vi "Read commandName.vi"(8 "error in (no error)":errorcluster, 11 "GoToStandby in":refnum<class "SetSpectTempSetpoint.lvclass">) -> (0 "error out":errorcluster, 2 "CommandValue":T1, 3 "GoToStandby out":refnum<class "SetSpectTempSetpoint.lvclass">)   [LabVIEW 2016, in "Commands.lvlib" / "SetSpectTempSetpoint.lvclass"]
uses:
  SetSpectTempSetpoint.lvclass
  Typedefs/CommandValue.ctl
  Typedefs/EXATypedefs.lvlib
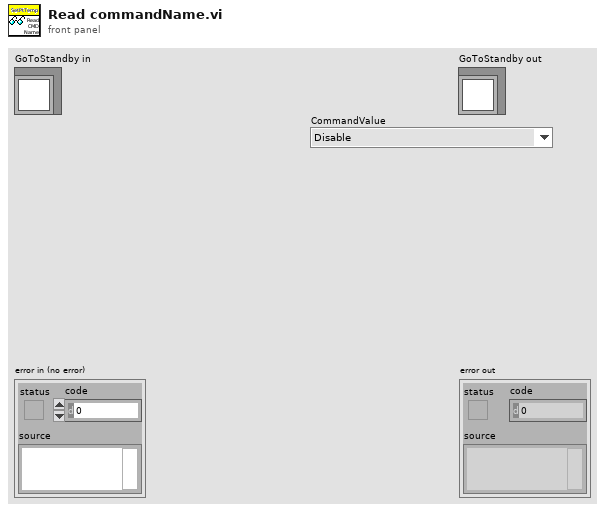
[diagram p1: front panel]
types:
  T1 = typedef "EXATypedefs.lvlib/CommandValue.ctl" = enum16{"Disable", "Enable", "Exit", "GoToStandby", "OnHeartbeat", "OnIncomingMessagingError", "OnInterrupt", "Start", "CaptureSpectImage", "SetSpectTempSetpoint", "StopImageCapture"}
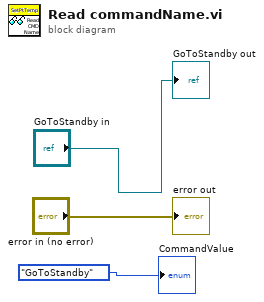
[diagram p0: block diagram]
diagram:
  "error out" <- "error in (no error)"
  "GoToStandby out" <- "GoToStandby in"
  "CommandValue" <- CommandValue."GoToStandby" ("CommandValue")
